vi "_Validate Method.vi"(7 "AcqMethod In":T1[](array[typedef]) {"ScanType" format="%#.6g"; "Mass Range"."Res" items=["High/High", "Medium/Medium", "Low/Low", "High/Medium", "High/Low", "Medium/High", "Medium/Low", "Low/High", "Low/Medium"]}) -> (0 "Expt List":string[](array[string]), 1 "Method Table":string[][](table), 2 "Run Duration (min)":dbl, 3 "AcqMethod Out":T1[](array[typedef]) {"ScanType" format="%#.6g"; "Mass Range"."Res" items=["High/High", "Medium/Medium", "Low/Low", "High/Medium", "High/Low", "Medium/High", "Medium/Low", "Low/High", "Low/Medium"]})   [LabVIEW 2012]
uses:
  Type/_XML Expt.ctl
  Type/_XML Lens.ctl
  Type/_Mass Range Property.ctl
  Type/_Mass Range Parameters.ctl
  Type/_RT Res Type.ctl
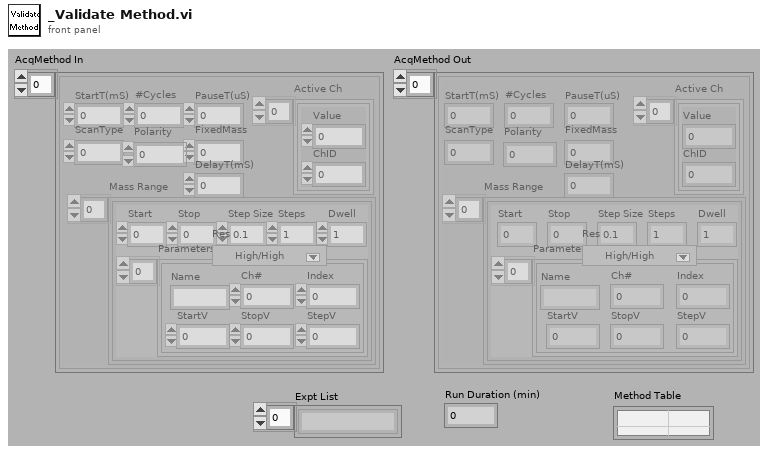
[diagram p1: front panel]
types:
  T1 = typedef "_XML Expt.ctl" = cluster{"StartT(mS)":i32, "#Cycles":i32, "PauseT(uS)":i32, "ScanType":i32, "Polarity":u8, "FixedMass":dbl, "DelayT(mS)":i32, "Active Ch":T2[], "Mass Range":T3[]}
  T2 = typedef "_XML Lens.ctl" = cluster{"Value":dbl, "ChID":u8}
  T3 = typedef "_Mass Range Property.ctl" = cluster{"Start":dbl, "Stop":dbl, "Step Size":dbl, "Steps":i32, "Dwell":dbl, "Parameters":T4[], "Res":T5}
  T4 = typedef "_Mass Range Parameters.ctl" = cluster{"Name":string, "Ch#":u8, "StartV":dbl, "StopV":dbl, "StepV":dbl, "Index":u8}
  T5 = typedef "_RT Res Type.ctl" = u16
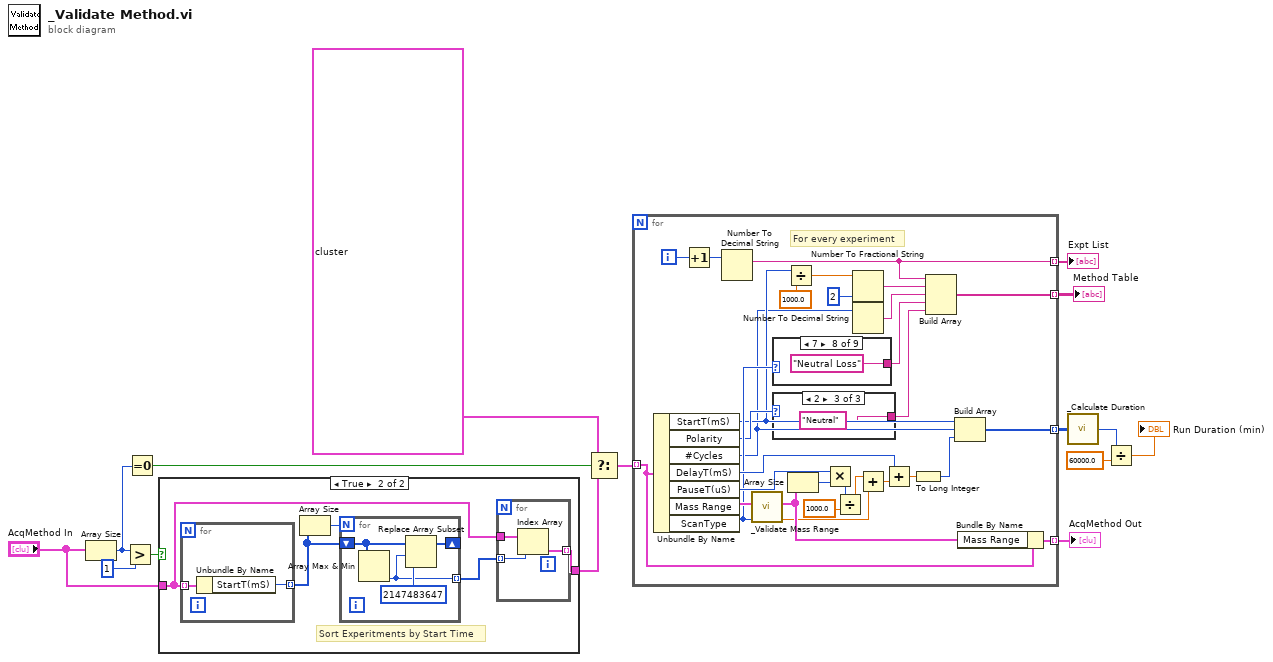
[diagram p0: block diagram]
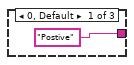
[diagram p2: hidden frame]
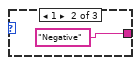
[diagram p3: hidden frame]
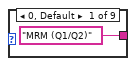
[diagram p4: hidden frame]
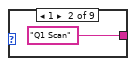
[diagram p5: hidden frame]
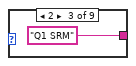
[diagram p6: hidden frame]
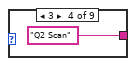
[diagram p7: hidden frame]
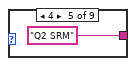
[diagram p8: hidden frame]
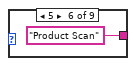
[diagram p9: hidden frame]
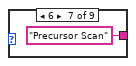
[diagram p10: hidden frame]
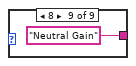
[diagram p11: hidden frame]
diagram:
  n1 = Array Size(array="AcqMethod In") -> (size(s)=w12:i32)
  n2 = Greater?(x=w12, y=1) -> (0:w13:bool)
  n3 = Equal To 0?(x=w12) -> (x = 0?=w11:bool)
  n4 = case shown="True" w13 {
    tunnel: "AcqMethod In" -> [w16 w18]
    tunnel: [w16 w17] -> w10
    frame False {
    }
    frame True {
      # "Sort Experitments by Start Time"
      n5 = for {
        tunnel: w18 -> [w30] mode=indexing
        tunnel: [w29] -> w20 mode=indexing
        n6 = Unbundle By Name(w30) -> ("StartT(mS)"=w29:i32)
      }
      n7 = Array Size(array=w20) -> (size(s)=w21:i32)
      n8 = for {
        N: w21 -> [_]
        shift-right: [w27] -> _
        shift-left: w20 -> [w28]
        tunnel: [w25] -> w19 mode=indexing
        n9 = Array Max & Min(array=w28) -> (min index (indices)=w25:i32)  [unwired: 3 out]
        n10 = Replace Array Subset(array=w28, new element=2147483647 ("new element/subarray"), index=w25) -> (w27:i32[])
      }
      n11 = for {
        tunnel: w19 -> [w24] mode=indexing
        tunnel: w18 -> [w23]
        tunnel: [w22] -> w17 mode=indexing
        n12 = Index Array(array=w23, index=w24) -> (element=w22:T1)
      }
    }
  }
  n13 = Select(t=T1[] [{"StartT(mS)"=0, "#Cycles"=100, "PauseT(uS)"=0, "ScanType"=1, "Polarity"=0, "FixedMass"=100.0, "DelayT(mS)"=0, "Active Ch"=[], "Mass Range"=[{"Start"=100.0, "Stop"=200.0, "Step Size"=0.1, "Steps"=1001, "Dwell"=1.0, "Parameters"=[], "Res"=0}]}] ("AcqMethod"), s=w11, f=w10) -> (s? t:f=w8:T1[])
  n14 = for {
    tunnel: w8 -> [w59] mode=indexing
    tunnel: [w52] -> w7 mode=indexing
    tunnel: [w46] -> w6 mode=indexing
    tunnel: [w37] -> w5 mode=indexing
    tunnel: [w31] -> w4 mode=indexing
    i -> [w43]
    # "For every experiment"
    n15 = Unbundle By Name(w59) -> ("StartT(mS)"=w34:i32, "Polarity"=w36:u8, "#Cycles"=w33:i32, "DelayT(mS)"=w53:i32, "PauseT(uS)"=w56:i32, "Mass Range"=w60:T3[], "ScanType"=w45:i32)
    n16 = Increment(x=w43) -> (x+1=w42:i32)
    n17 = Number To Decimal String(number=w42) -> (decimal integer string=w37:string)  [unwired: 1 out]
    n18 = call "_Validate Mass Range.vi"("Run Mode"=w45, "Mass Ranges"=w60) -> ("Cycle Time (ms)"=w55:dbl, "Mass Ranges Out"=w57:T3[])  [unwired: 2 in, 4 out]
    n19 = case shown="7" w45 {
      tunnel: ["MRM (Q1/Q2)" "Q1 Scan" "Q1 SRM" "Q2 Scan" "Q2 SRM" "Product Scan" "Precursor Scan" "Neutral Loss" "Neutral Gain"] -> w44
      frame 0, Default {
      }
      frame 1 {
      }
      frame 2 {
      }
      frame 3 {
      }
      frame 4 {
      }
      frame 5 {
      }
      frame 6 {
      }
      frame 7 {
      }
      frame 8 {
      }
    }
    n20 = case shown="2" w36 {
      tunnel: ["Postive" "Negative" "Neutral"] -> w35
      frame 0, Default {
      }
      frame 1 {
      }
      frame 2 {
      }
    }
    n21 = Divide(x=w34, y=1000.0) -> (x/y=w50:dbl)
    n22 = Array Size(array=w57) -> (size(s)=w58:i32)
    n23 = Multiply(x=w56, y=w58) -> (x*y=w39:i32)
    n24 = Divide(x=w39, y=1000.0) -> (x/y=w38:dbl)
    n25 = Number To Fractional String(number=w50, precision (6)=2) -> (F-format string=w48:string)  [unwired: 2 out]
    n26 = Number To Decimal String(number=w33) -> (decimal integer string=w47:string)  [unwired: 1 out]
    n27 = Add(x=w38, y=w55) -> (x+y=w54:dbl)
    n28 = Add(x=w53, y=w54) -> (x+y=w40:dbl)
    n29 = To Long Integer(number=w40) -> (32bit integer=w32:i32)
    n30 = Build Array(w37, w48, w47, w44, w35) -> (w46:string[])
    n31 = Build Array(w34, w33, w32) -> (w31:i32[])
    n32 = Bundle By Name(cluster=w59, "Mass Range"=w57) -> (w52:T1)
  }
  "AcqMethod Out" <- w7
  "Method Table" <- w6
  "Expt List" <- w5
  n33 = call "_Calculate Duration.vi"("Method"=w4) -> ("RunTime(mS)"=w3:i32)
  n34 = Divide(x=w3, y=60000.0) -> (x/y=→"Run Duration (min)":dbl)
